vi "PPMS temp set point.vi"(0 "GPIB address":string="15", 1 "error in (no error)":errorcluster) -> (2 "Temperature set point (K)":dbl format="%.2f", 3 "Set rate (K/min)":dbl format="%.2f", 4 "error out":errorcluster)   [LabVIEW 2018]
doc: "This VI returns the set temperature of the PPMS system and the set rate of change of the temperature. Note that this is not necessarily the actual temperature, it is just what the PPMS is going towards."
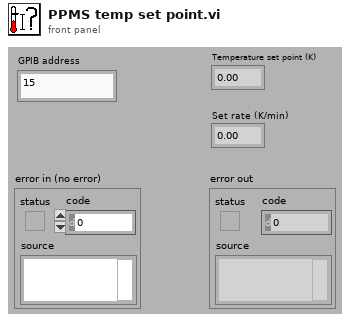
[diagram p1: front panel]
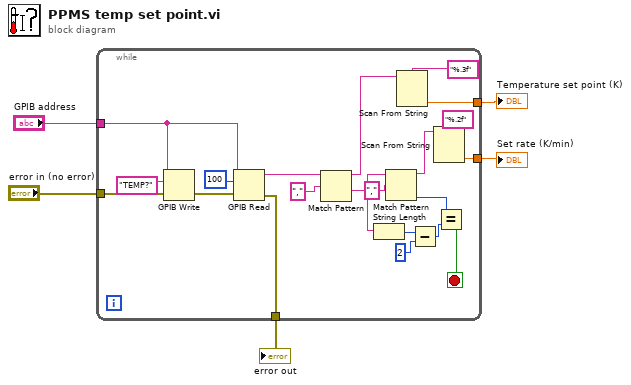
[diagram p0: block diagram]
diagram:
  n1 = while {
    tunnel: "GPIB address" -> [w26]
    tunnel: "error in (no error)" -> [w25]
    tunnel: [w23] -> w3
    tunnel: [w18] -> w2
    tunnel: [w13] -> w1
    stop <- w6 stop-if-true
    n2 = GPIB Write(0:w26, 1:"TEMP?", 3:w25) -> (6:w24:errorcluster)  [unwired: 3 out]
    n3 = GPIB Read(0:w26, 1:100, 3:w24) -> (5:w20:string, 7:w23:errorcluster)  [unwired: 3 out]
    n4 = Match Pattern(string=w20, regular expression=",") -> (before substring=w15:string, after substring=w11:string)  [unwired: 3 out]
    n5 = String Length(string=w11) -> (length=w8:i32)
    n6 = Match Pattern(string=w11, regular expression=",") -> (before substring=w14:string, offset past match=w10:i32)  [unwired: 3 out]
    n7 = Scan From String(format string="%.3f", input string=w15) -> (output 1=w18:dbl)  [unwired: 2 in, 4 out]
    n8 = Subtract(x=w8, y=2) -> (x-y=w9:i32)
    n9 = Scan From String(format string="%.2f", input string=w14) -> (output 1=w13:dbl)  [unwired: 2 in, 4 out]
    n10 = Equal?(x=w10, y=w9) -> (x = y?=w6:bool)
  }
  "error out" <- w3
  "Temperature set point (K)" <- w2
  "Set rate (K/min)" <- w1
